vi "Waveform Simulator_MyApplication.vi"() -> ()   [LabVIEW 2017]
uses:
  <vilib>/imath/engines/lvmath2/RunTimeEngine/Managers/WorkSpace/UID Generator.vi
  <vilib>/imath/engines/lvmath2/RunTimeEngine/RunTimeType/NIMS_RunTimeType_From StrictType (excl LVString).vi
  <instcachedir>/0/NIMS_RunTimeType_From StrictType (excl LVString)_1019F277F0A747EDBCA0F6C52CA54500.lvgen/NIMS_RunTimeType_From StrictType (excl LVString)_1019F277F0A747EDBCA0F6C52CA54500_000.vi
  <vilib>/imath/engines/lvmath2/RunTimeEngine/LocalVariableDefStatement/MC_LocalVariableDefStatement_Display.vi
  <vilib>/imath/engines/lvmath2/RunTimeEngine/RangeToken/NIMS_Range.vi
  <instcachedir>/0/NIMS_Range_69CB9AAD882742A19CF7E739BE79952C.lvgen/NIMS_Range_69CB9AAD882742A19CF7E739BE79952C_000.vi
  <vilib>/imathl/engines/lvmath/Functions/Error Handling/Create Error.vi
  <vilib>/imath/engines/lvmath2/RunTimeEngine/Managers/SymbolTable/Clear UID.vi
  <vilib>/imath/engines/lvmath2/RunTimeEngine/NodeEndStatement/NIMS_NodeEndStatement_Output.vi
  <instcachedir>/0/NIMS_NodeEndStatement_Output_53EC0D466D134D7ABD903AC30B43404B.lvgen/NIMS_NodeEndStatement_Output_53EC0D466D134D7ABD903AC30B43404B_005.vi
  <vilib>/imath/engines/lvmath2/RunTimeEngine/ErrorHandling/NIMS_Finalize Error.vi
  <vilib>/imath/engines/lvmath2/RunTimeEngine/Managers/SymbolTable/NIMS_WorkSpace.lvlib
panel:
  out "Waveform Graph":dbl[](graph)
  out "element":dbl
  in  "stop":bool
  out "Waveform Chart":dbl(graph)
  out "XY Graph 2":cluster{"t1":dbl[], "lambda1":dbl[]}(graph)
  out "size(s)":i32
  out "output array":dbl[](array[numeric])
  in  "Sampling Frequency2":dbl=1000.0
  in  "BreakTime":dbl
  in  "One Cycle":dbl=10.0
  in  "Max Contraction Ratio":dbl=0.3
  in  "Initial Contraction Ratio":dbl=0.1
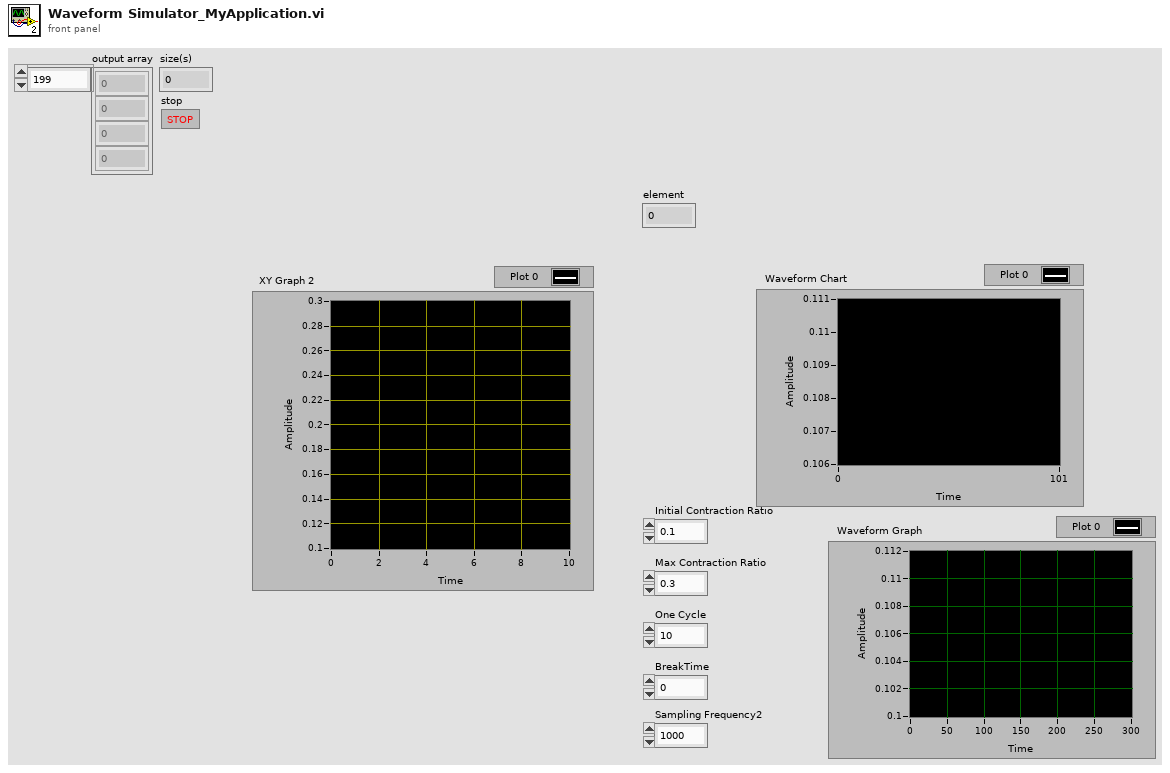
[diagram p1: front panel]
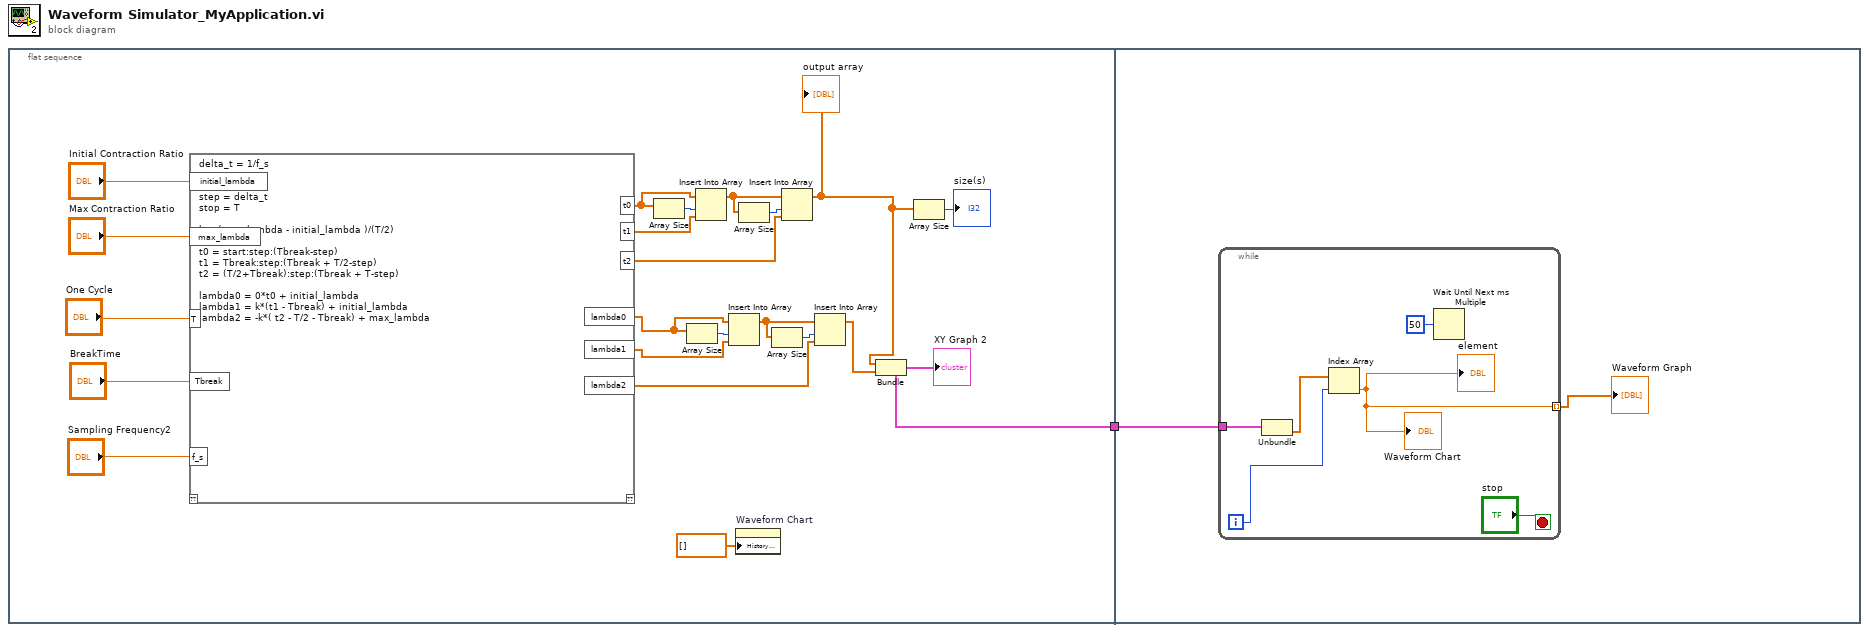
[diagram p0: block diagram]
diagram:
  n1 = flat-sequence {
    tunnel: [w17] -> w1
    tunnel: w1 -> [w283]
    frame #0 {
      n2 = mathscript code="delta_t = 1/f_s\n\nstart = 0\nstep = delta_t\nstop = T\n\nk = (max_lambda - initial_lambda )/(T/2)\n\nt0 = start:step:(Tbreak-step)\nt1 = Tbreak:step:(Tbreak + T/2-step)\nt2 = (T/2+Tbreak):step:(Tbreak + T-step)\n\nlambda0 = 0*t0 + initial_lambda\nlambda1 = k*(t1 - Tbreak) + initial_lambda\nlambda2 = -k*( t2 - T/2 - Tbreak) + max_lambda"("initial_lambda"="Initial Contraction Ratio", "max_lambda"="Max Contraction Ratio", "T"="One Cycle", "f_s"="Sampling Frequency2", "Tbreak"="BreakTime") -> ("t1"=w13:dbl[], "t2"=w12:dbl[], "lambda1"=w4:dbl[], "lambda2"=w3:dbl[], "t0"=w14:dbl[], "lambda0"=w5:dbl[])  [unwired: 1 in, 1 out]
      n3 = Array Size(array=w14) -> (size(s)=w19:i32)
      n4 = Array Size(array=w5) -> (size(s)=w6:i32)
      n5 = Insert Into Array(array=w14, index=w19, new element=w13) -> (w10:dbl[])
      n6 = Insert Into Array(array=w5, index=w6, new element=w4) -> (w8:dbl[])
      n7 = property on="Waveform Chart" class="WFChart (strict)"("History Data"=dbl[] []) -> ()  [unwired: 2 in, 2 out]
      n8 = Array Size(array=w10) -> (size(s)=w11:i32)
      n9 = Array Size(array=w8) -> (size(s)=w7:i32)
      n10 = Insert Into Array(array=w10, index=w11, new element=w12) -> (w9:dbl[])
      "output array" <- w9
      n11 = Insert Into Array(array=w8, index=w7, new element=w3) -> (w2:dbl[])
      n12 = Bundle("t0"=w9, "lambda0"=w2) -> (w17:cluster{"t0":dbl[], "lambda0":dbl[]})  [unwired: 1 in]
      "XY Graph 2" <- w17
      n13 = Array Size(array=w9) -> (size(s)=→"size(s)":i32)
    }
    frame #1 {
      n14 = while {
        tunnel: w283 -> [w289]
        tunnel: [w284] -> w282 mode=indexing
        i -> [w285]
        stop <- "stop" stop-if-true
        n15 = Unbundle(w289) -> ("lambda0"=w286:dbl[])  [unwired: 1 out]
        n16 = Index Array(array=w286, index=w285) -> (element=w284:dbl)
        "Waveform Chart" <- w284
        "element" <- w284
        n17 = Wait Until Next ms Multiple(millisecond multiple=u32 50) -> ()  [unwired: 1 out]
      }
      "Waveform Graph" <- w282
    }
  }
